vi "V to R.vi"(8 "Reference R(k)":dbl, 10 "Voltage output":dbl, 11 "Measured V":dbl) -> (3 "Themistor R":dbl)   [LabVIEW 2019]
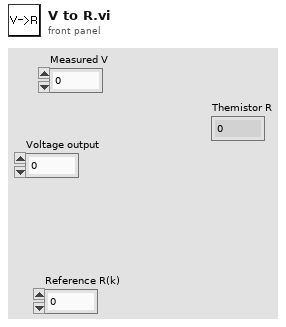
[diagram p1: front panel]
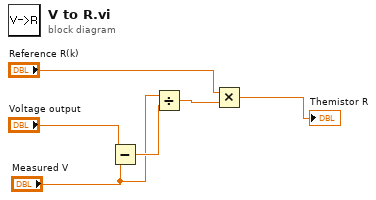
[diagram p0: block diagram]
diagram:
  n1 = Subtract(x="Voltage output", y="Measured V") -> (x-y=w3:dbl)
  n2 = Divide(x="Measured V", y=w3) -> (x/y=w4:dbl)
  n3 = Multiply(x="Reference R(k)", y=w4) -> (x*y=→"Themistor R":dbl)
